vi "GetPositionDelta.vi"(7 "Move Vector":T1, 8 "error in (no error)":errorcluster, 10 "Yaw":sgl, 11 "3D Scene in":refnum<class "3D Scene.lvclass">) -> (0 "error out":errorcluster, 2 "Position Delta":cluster{"X":sgl, "Y":sgl, "Z":sgl}, 3 "3D Scene out":refnum<class "3D Scene.lvclass">)   [LabVIEW 2015, in "3D Scene.lvclass"]
uses:
  3D Scene.lvclass
  3D Point.ctl
  <vilib>/Analysis/baseanly.llb/Vector x A.vi
  <vilib>/Analysis/NI_AALBase.lvlib
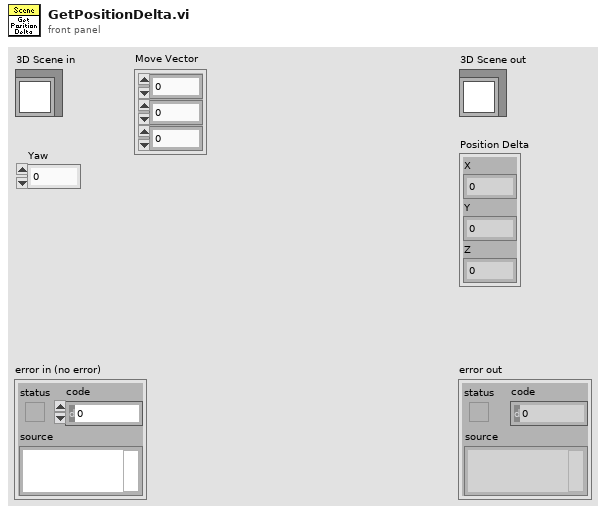
[diagram p1: front panel]
types:
  T1 = typedef "3D Point.ctl" = cluster{"X":sgl, "Y":sgl, "Z":sgl}
  T2 = typedef "NI_Matrix.lvlib/RealMatrix.ctl" = dbl[][]
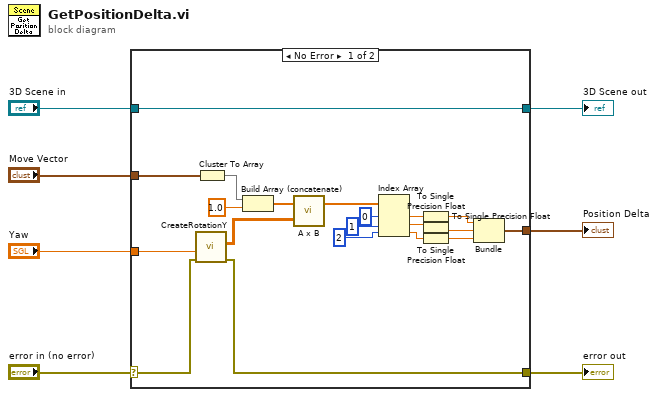
[diagram p0: block diagram]
diagram:
  n1 = case shown="No Error" "error in (no error)" {
    selector: "error in (no error)" -> [w20 w29]
    tunnel: [w19 w29] -> w6
    tunnel: [w27 w28] -> w4
    tunnel: "3D Scene in" -> [w27 w28]
    tunnel: "Move Vector" -> [w22 _]
    tunnel: "Yaw" -> [w21 _]
    tunnel: [w15 _] -> w1
    frame No Error {
      n2 = call "CreateRotationY.vi"("error in (no error)"=w20, "radians"=w21) -> ("error out"=w19:errorcluster, "modelview rotated"=w23:T2)  [unwired: 7 in, 1 out]
      n3 = Cluster To Array(cluster=w22) -> (array=w25:sgl[])
      n4 = Build Array (concatenate)(w25, sgl 1.0 ("element")) -> (w24:sgl[])
      n5 = call-poly <vilib>:"A x B.vi"("Matrix A"=w23, "Vector V'"=w24) -> ("V' x A"=w18:dbl[])  [unwired: 1 out]
      n6 = Index Array(array=w18, index #1=0 ("index"), index #2=1 ("index"), index #3=2 ("index")) -> (element #1=w17:dbl, element #2=w14:dbl, element #3=w13:dbl)
      n7 = To Single Precision Float(number=w17) -> (single precision float=w16:sgl)
      n8 = To Single Precision Float(number=w14) -> (single precision float=w12:sgl)
      n9 = To Single Precision Float(number=w13) -> (single precision float=w11:sgl)
      n10 = Bundle(w16, w12, w11) -> (w15:cluster{sgl, sgl, sgl})  [unwired: 1 in]
    }
    frame Error {
    }
  }
  "error out" <- w6
  "3D Scene out" <- w4
  "Position Delta" <- w1
